vi "FEMTO_Gain.vi"(10 "Femto Gain In V/A":refnum<vi>) -> ()   [LabVIEW 2025]
uses:
  <userlib>/_FEMTO Messtechnik GmbH/LUCI-10/_TypeDefs/Choose_Device_Enum.ctl
  <userlib>/_FEMTO Messtechnik GmbH/LUCI-10/Control/Set_Gain_DLPCA-200.vi
  <userlib>/_FEMTO Messtechnik GmbH/LUCI-10/FEMTO_LUCI-10.lvlib
panel:
  in  "Femto Gain V/A":dbl(ring) items=["1E3"=1.0, "1E4"=2.0, "1E5"=3.0, "1E6"=4.0, "1E7"=5.0, "1E8"=6.0, "1E9"=7.0]
  out "Numeric":dbl
  in  "Available LUCI-10 Devices":i32(listbox)
  in  "Info":bool
  out "Overload":bool
  in  "Rahmen":bool
  in  "stop":bool
  out "LED":bool
  in  "Check LUCI":bool
  out "String_Product":string
  in  "Product_String":bool
  # "Remote Control LUCI-10 DLPCA-200"
  # "DLPCA-200"
  # "Configuration"
  # "Gain Setting"
  # "5"
  # "6"
  # "7"
  # "8"
  # "9"
  # "10"
  # "11"
  # "10"
  # "10"
  # "10"
  # "10"
  # "10"
  # "10"
  # "10"
  # "H"
  # "V/A"
  # "Device Information"
  # "L"
  # "3"
  # "4"
  # "5"
  # "6"
  # "7"
  # "8"
  # "9"
  # "10"
  # "10"
  # "10"
  # "10"
  # "10"
  # "10"
  # "10"
  # "500"
  # "500"
  # "400"
  # "200"
  # "50"
  # "7"
  # "1"
  # "kHz"
  # "Overload"
  # "Coupling"
  # "AC"
  # "DC"
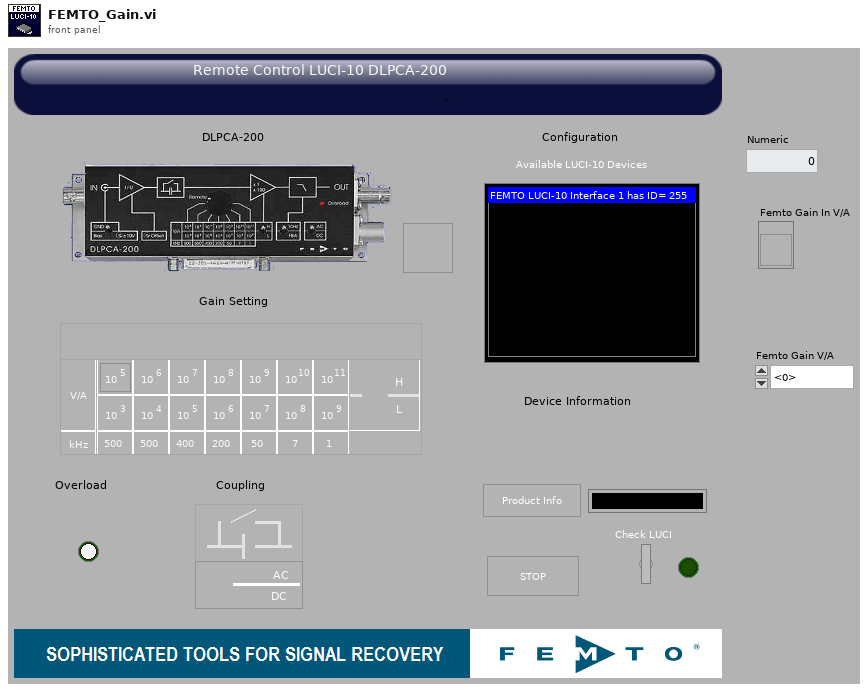
[diagram p1: front panel]
types:
  T1 = typedef "FEMTO_LUCI-10.lvlib/Choose_Device_Enum.ctl" = enum16{"DDPCA-300", "DLPCA-200", "DHPCA-100", "OE-200", "OE-300", "LIA-MV-150-S", "LIA-MV-150-D", "LIA-MV-200-L", "LIA-MV-200-H", "LIA-MVD-200-L", "LIA-MVD-200-H", "DLPVA-100-BUN-S", "DLPVA-100-BLN-S", "DLPVA-100-B-S", "DLPVA-100-B-D", "DLPVA-100-F-S", "DLPVA-100-F-D", "DHPVA-100", "DHPVA-200", "DUPVA-1-60", "DUPVA-1-70"}
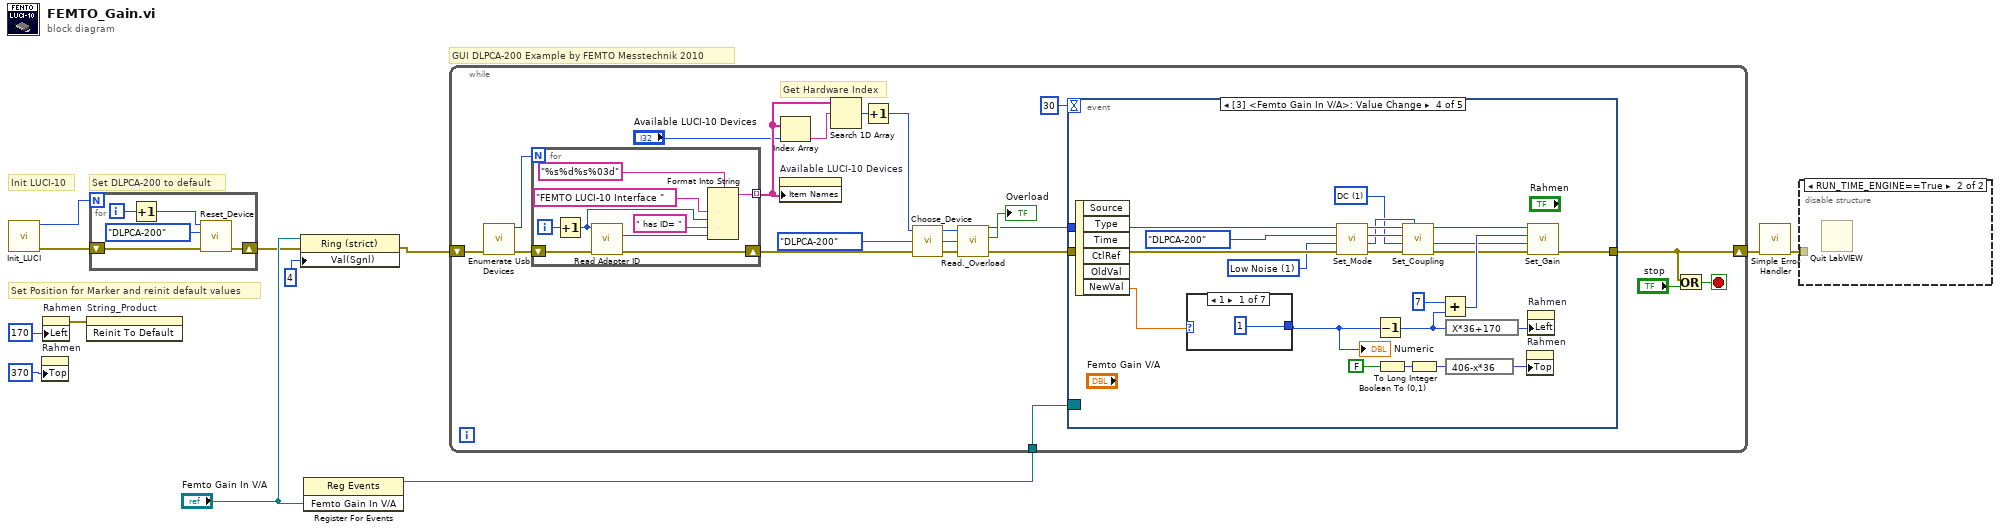
[diagram p0: block diagram]
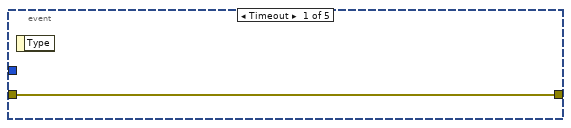
[diagram p3: hidden frame]
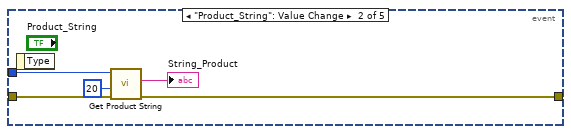
[diagram p4: hidden frame]
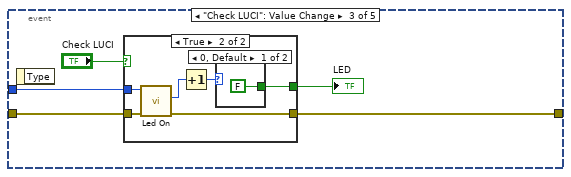
[diagram p5: hidden frame]
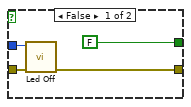
[diagram p6: hidden frame]
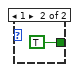
[diagram p7: hidden frame]
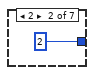
[diagram p8: hidden frame]
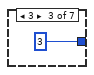
[diagram p9: hidden frame]
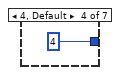
[diagram p10: hidden frame]
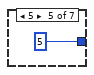
[diagram p11: hidden frame]
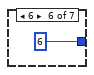
[diagram p12: hidden frame]
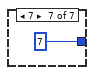
[diagram p13: hidden frame]
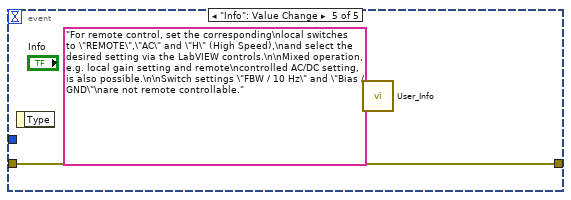
[diagram p14: hidden frame]
diagram:
  # "Set DLPCA-200 to default"
  # "Set Position for Marker and reinit default values"
  # "Init LUCI-10"
  # "GUI DLPCA-200 Example by FEMTO Messtechnik 2010"
  n1 = call <userlib>:"Init_LUCI.vi"() -> ("error out"=w9:errorcluster, "Number of Devices"=w10:i32)  [unwired: 10 in]
  n2 = property on="Rahmen" class="Bool"("Top"=370 ("Position:Top")) -> ()  [unwired: 2 in, 2 out]
  n3 = property on="Rahmen" class="Bool"("Left"=170 ("Position:Left")) -> (error out=w8:errorcluster)  [unwired: 2 in, 1 out]
  n4 = invoke on="String_Product" class="Str" method="Reinit To Default"(error in=w8) -> ()  [unwired: 2 in, 3 out]
  n5 = for {
    N: w10 -> [_]
    shift-right: [w13] -> w2
    shift-left: w9 -> [w14]
    i -> [w17]
    n6 = Increment(x=w17) -> (x+1=w15:i32)
    n7 = call <userlib>:"Reset_Device.vi"("error in (no error)"=w14, "Choose_Device"=Choose_Device_Enum."DLPCA-200", "Index"=w15) -> ("error out"=w13:errorcluster)  [unwired: 4 in, 2 out]
  }
  n8 = property class="Ring (strict)"(reference="Femto Gain In V/A", error in=w2, "Val(Sgnl)"=4) -> (error out=w1:errorcluster)  [unwired: 1 out]
  n9 = register-events("Femto Gain In V/A") -> (reference out=w5:refnum<event-registration>)  [unwired: 2 in, 1 out]
  n10 = while {
    shift-right: [w19] -> w7
    shift-left: w1 -> [w28]
    tunnel: w5 -> [w18]
    stop <- w20 stop-if-true
    # "Get Hardware Index"
    n11 = call <userlib>:"Enumerate Usb Devices.vi"("error in (no error)"=w28) -> ("error out"=w21:errorcluster, "function return"=w29:i32)  [unwired: 9 in]
    n12 = for {
      N: w29 -> [_]
      tunnel: [w41] -> w25 mode=indexing
      shift-right: [w40] -> w22
      shift-left: w21 -> [w39]
      i -> [w42]
      n13 = Increment(x=w42) -> (x+1=w47:i32)
      n14 = call <userlib>:"Read Adapter ID.vi"("error in (no error)"=w39, "index"=w47) -> ("error out"=w40:errorcluster, "id out"=w46:i32)  [unwired: 7 in, 1 out]
      n15 = Format Into String(format string="%s%d%s%03d", "FEMTO LUCI-10 Interface ", w47, " has ID= ", w46) -> (resulting string=w41:string)  [unwired: 2 in, 1 out]
    }
    n16 = property on="Available LUCI-10 Devices" class="LstBox (strict)"("Item Names"=w25) -> ()  [unwired: 2 in, 2 out]
    n17 = Index Array(array=w25, index="Available LUCI-10 Devices") -> (element=w26:string)
    n18 = Search 1D Array(1D array=w25, element=w26) -> (index of element=w27:i32)  [unwired: 1 in]
    n19 = Increment(x=w27) -> (x+1=w23:i32)
    n20 = call <userlib>:"Choose_Device.vi"("error in (no error)"=w22, "Choose_Device"=Choose_Device_Enum."DLPCA-200", "Index"=w23) -> ("error out"=w34:errorcluster, "Device_type"=w35:T1, "Index_Out"=w36:i32)
    n21 = call <userlib>:"Read._Overload.vi"("Index"=w36, "Choose_Device"=w35, "error in (no error)"=w34) -> ("Index_Out"=w30:i32, "Overload"=→"Overload":bool, "error out"=w31:errorcluster)  [unwired: 1 out]
    n22 = event shown="[3] <Femto Gain In V/A>: Value Change" {
      selector: w18 -> [_ _ _ _ _]
      dyn-events: _ -> [_ _ _ _ _]
      timeout: 30 -> [_ _ _ _ _]
      tunnel: w31 -> [w48 w51 w56 w78 w101]
      tunnel: w30 -> [_ w53 w57 w89 _]
      tunnel: [w48 w49 w54 w76 w101] -> w19
      event Timeout {
        n23 = event-data() -> ()  [unwired: 1 in, 1 out]
      }
      event "Product_String": Value Change {
        n24 = event-data() -> ()  [unwired: 1 in, 1 out]
        n25 = call <userlib>:"Get Product String.vi"("error in (no error)"=w51, "size"=20, "index"=w53) -> ("error out"=w49:errorcluster, "string out"=→"String_Product":string)  [unwired: 6 in, 1 out]
      }
      event "Check LUCI": Value Change {
        n26 = event-data() -> ()  [unwired: 1 in, 1 out]
        n27 = case shown="True" "Check LUCI" {
          tunnel: w57 -> [w62 w68]
          tunnel: w56 -> [w61 w67]
          tunnel: [FALSE w64] -> w55
          tunnel: [w59 w63] -> w54
          frame False {
            n28 = call <userlib>:"Led Off.vi"("error in (no error)"=w61, "index"=w62) -> ("error out"=w59:errorcluster)  [unwired: 8 in, 1 out]
          }
          frame True {
            n29 = call <userlib>:"Led On.vi"("error in (no error)"=w67, "index"=w68) -> ("error out"=w63:errorcluster, "function_return"=w66:i32)  [unwired: 7 in, 1 out]
            n30 = Increment(x=w66) -> (x+1=w65:i32)
            n31 = case shown="0, Default" w65 {
              tunnel: [FALSE TRUE] -> w64
              frame 0, Default {
              }
              frame 1 {
              }
            }
          }
        }
        "LED" <- w55
      }
      event Value Change {
        w75 = u16 1 items=["AC", "DC"] ("Set Coupling")
        w73 = u16 1 items=["High Speed", "Low Noise"] ("Set Mode")
        n32 = event-data() -> ("NewVal"=w71:dbl)  [unwired: 1 in, 5 out]
        n33 = case shown="1" w71 {
          tunnel: [1 2 3 4 5 6 7] -> w72
          frame 1 {
          }
          frame 2 {
          }
          frame 3 {
          }
          frame 4, Default {
          }
          frame 5 {
          }
          frame 6 {
          }
          frame 7 {
          }
        }
        "Numeric" <- w72
        n34 = call <userlib>:"Set_Mode.vi"("error in (no error)"=w78, "Set Mode"=w73, "Choose_Device"=Choose_Device_Enum."DLPCA-200", "Index"=w89) -> ("error out"=w83:errorcluster, "Status_out"=w84:i32, "Device_type"=w85:T1, "Index_Out"=w86:i32)  [unwired: 1 in]
        n35 = Decrement(x=w72) -> (x-1=w87:i32)
        n36 = Boolean To (0,1)(Boolean=FALSE) -> (0, 1=w93:i16)
        n37 = call <userlib>:"Set_Coupling.vi"("Status"=w84, "error in (no error)"=w83, "Set Coupling"=w75, "Choose_Device"=w85, "Index"=w86) -> ("error out"=w79:errorcluster, "Status_out"=w80:i32, "Index_Out"=w82:i32)  [unwired: 1 out]
        n38 = To Long Integer(number=w93) -> (32bit integer=w92:i32)
        n39 = Add(x=7, y=w87) -> (x+y=w81:i32)
        n40 = expression code="X*36+170"(w87) -> (w91:i32)
        n41 = expression code="406-x*36"(w92) -> (w90:i32)
        n42 = property on="Rahmen" class="Bool"("Top"=w90) -> ()  [unwired: 2 in, 2 out]
        n43 = call-poly <userlib>:"Set_Gain.vi"("error in"=w79, "Status"=w80, "Gain  [V/A]"=w81, "index"=w82) -> ("error out"=w76:errorcluster)  [unwired: 2 out]
        n44 = property on="Rahmen" class="Bool"("Left"=w91) -> ()  [unwired: 2 in, 2 out]
      }
      event "Info": Value Change {
        n45 = event-data() -> ()  [unwired: 1 in, 1 out]
        n46 = call <userlib>:"User_Info.vi"("String"="For remote control, set the corresponding\nlocal switches to \"REMOTE\",\"AC\" and \"H\" (High Speed),\nand select the desired setting via the LabVIEW controls.\n\nMixed operation, e.g. local gain setting and remote\ncontrolled AC/DC setting, is also possible.\n\nSwitch settings \"FBW / 10 Hz\" and \"Bias / GND\"\nare not remote controllable.") -> ()  [unwired: 1 in]
      }
    }
    n47 = Or(x=w19, y="stop") -> (x .or. y?=w20:bool)
  }
  n48 = call <vilib>:"Simple Error Handler.vi"("error in (no error)"=w7) -> ("error out"=w6:errorcluster)  [unwired: 4 in, 4 out]
  n49 = disable-structure shown="RUN_TIME_ENGINE==True" {
    disable-tunnel: w6 -> [_ _]
    frame condition #0 (active) {
    }
    frame condition #1 {
      n50 = Quit LabVIEW() -> ()  [unwired: 1 in]
    }
  }
